vi "ProcessCurveData.vi"(11 "New Curve Values":T1) -> ()   [LabVIEW 2025]
uses:
  NewCurveDataEventArgs.ctl
  E:/PSCode/PalmSens_SDK/labview/PalmSens/Libraries/PalmSens.Core.Simplified.LabVIEW.dll
  Libraries/PalmSens.Core.Simplified.LabVIEW.dll
  LiveCurveResult.ctl
  MeasurementsResult.ctl
  MeasurementResults.ctl
  CurvesByMeasurement.ctl
  MeasurementInfo.ctl
  CurveInfo.ctl
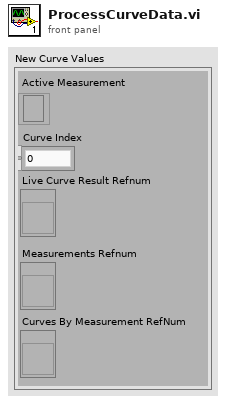
[diagram p1: front panel]
types:
  T1 = typedef "NewCurveDataEventArgs.ctl" = cluster{"Active Measurement":refnum<k24>, "Live Curve Result Refnum":refnum<vi>, "Measurements Refnum":refnum<vi>, "Curves By Measurement RefNum":refnum<vi>, "Curve Index":i32}
  T2 = typedef "CurvesByMeasurement.ctl" = map{refnum<k24>, T3}
  T3 = typedef "MeasurementInfo.ctl" = cluster{"Index":i32, "Is Measuring Refnum":refnum<vi>, "MeasurementEnded callback refnum":refnum<k27>, "SimpleCurveAdded callback refnum":refnum<k27>, "Live Curve Result Refnum":refnum<vi>, "Map":map{i32, T4}}
  T4 = typedef "CurveInfo.ctl" = cluster{"NewDataAdded callback refnum":refnum<k27>, "CurveFinished callback refnum":refnum<k27>}
  T5 = typedef "MeasurementsResult.ctl" = cluster{"Name":string, "Curves":T6, "Index":i32}[]
  T6 = typedef "MeasurementResults.ctl" = T7[]
  T7 = typedef "LiveCurveResult.ctl" = cluster{"X Label":string, "Y Label":string, "Name":string, "Index":i16, "Curve Values":cluster{"Values":cluster{"X Value":dbl, "Y Value":dbl}[], "Index":i16}}
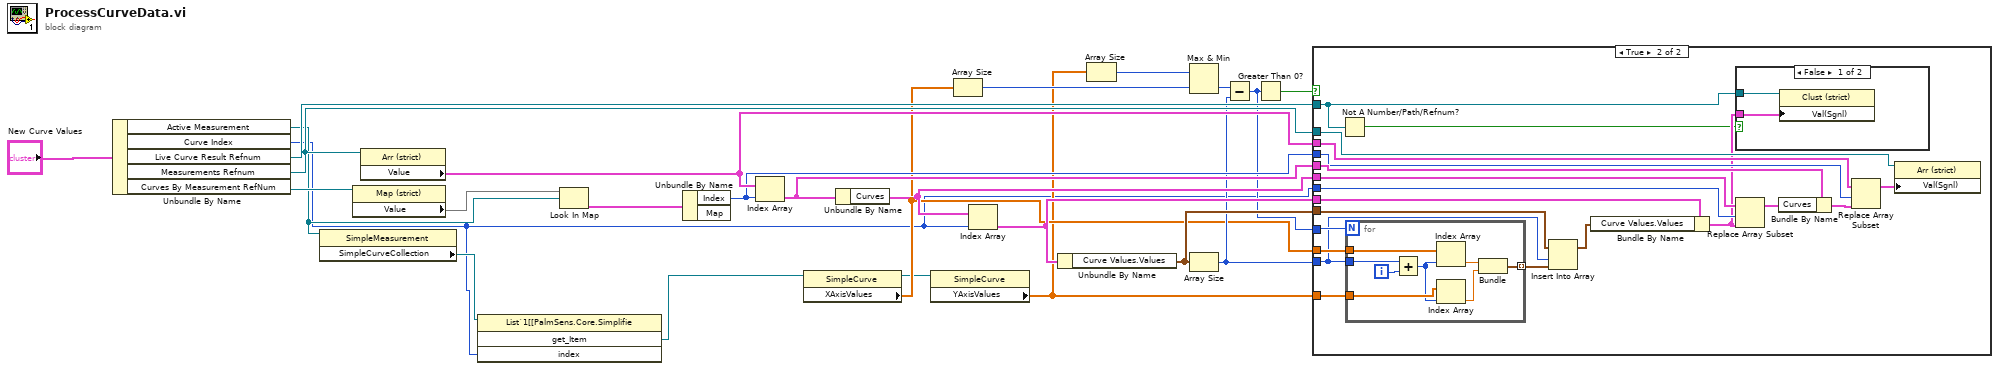
[diagram p0: block diagram]
diagram:
  n1 = Unbundle By Name("New Curve Values") -> ("Active Measurement"=w4:refnum<k24>, "Curve Index"=w2:i32, "Live Curve Result Refnum"=w21:refnum<vi>, "Measurements Refnum"=w25:refnum<vi>, "Curves By Measurement RefNum"=w9:refnum<vi>)
  n2 = property class="SimpleMeasurement"(reference=w4) -> ("SimpleCurveCollection"=w3:refnum<k24>)  [unwired: 1 in, 2 out]
  n3 = property class="Map (strict)"(reference=w9) -> ("Value"=w10:T2)  [unwired: 1 in, 2 out]
  n4 = property class="Arr (strict)"(reference=w25) -> ("Value"=w24:T5)  [unwired: 1 in, 2 out]
  n5 = invoke class="List`1[[PalmSens.Core.Simplifie" method="get_Item"(reference=w3, "index"=w2) -> ("get_Item"=w1:refnum<k24>)  [unwired: 2 in, 3 out]
  n6 = Look In Map(map=w10, key=w4) -> (value=w11:T3)  [unwired: 1 in, 1 out]
  n7 = Unbundle By Name(w11) -> ("Index"=w23:i32)  [unwired: 1 out]
  n8 = Index Array(array=w24, index=w23) -> (element=w22:cluster{"Name":string, "Curves":T6, "Index":i32})
  n9 = property class="SimpleCurve"(reference=w1) -> (reference out=w5:refnum<k24>, "XAxisValues"=w12:dbl[])  [unwired: 1 in, 1 out]
  n10 = Unbundle By Name(w22) -> ("Curves"=w20:T6)
  n11 = property class="SimpleCurve"(reference=w5) -> ("YAxisValues"=w7:dbl[])  [unwired: 1 in, 2 out]
  n12 = Array Size(array=w12) -> (size(s)=w13:i32)
  n13 = Index Array(array=w20, index=w2) -> (element=w19:T7)
  n14 = Unbundle By Name(w19) -> ("Curve Values.Values"=w18:cluster{"X Value":dbl, "Y Value":dbl}[])
  n15 = Array Size(array=w7) -> (size(s)=w6:i32)
  n16 = Max & Min(x=w6, y=w13) -> (min(x,y)=w14:i32)  [unwired: 1 out]
  n17 = Array Size(array=w18) -> (size(s)=w17:i32)
  n18 = Subtract(x=w14, y=w17) -> (x-y=w16:i32)
  n19 = Greater Than 0?(x=w16) -> (x > 0?=w15:bool)
  n20 = case shown="True" w15 {
    tunnel: w12 -> [_ w45]
    tunnel: w7 -> [_ w44]
    tunnel: w16 -> [_ w43]
    tunnel: w17 -> [_ w41]
    tunnel: w18 -> [_ w42]
    tunnel: w19 -> [_ w38]
    tunnel: w20 -> [_ w37]
    tunnel: w2 -> [_ w36]
    tunnel: w21 -> [_ w26]
    tunnel: w22 -> [_ w35]
    tunnel: w23 -> [_ w32]
    tunnel: w24 -> [_ w31]
    tunnel: w25 -> [_ w29]
    frame False {
    }
    frame True {
      n21 = Not A Number/Path/Refnum?(number/path/refnum=w26) -> (NaN/Path/Refnum?=w27:bool)
      n22 = for {
        N: w43 -> [_]
        tunnel: w45 -> [w55]
        tunnel: w44 -> [w52]
        tunnel: [w49] -> w40 mode=indexing
        tunnel: w41 -> [w48]
        i -> [w54]
        n23 = Add(x=w48, y=w54) -> (x+y=w51:i32)
        n24 = Index Array(array=w55, index=w51) -> (element=w53:dbl)
        n25 = Index Array(array=w52, index=w51) -> (element=w50:dbl)
        n26 = Bundle(w53, w50) -> (w49:cluster{dbl, dbl})  [unwired: 1 in]
      }
      n27 = Insert Into Array(array=w42, index=w41, new element=w40) -> (w39:cluster{"X Value":dbl, "Y Value":dbl}[])
      n28 = Bundle By Name(cluster=w38, "Curve Values.Values"=w39) -> (w28:T7)
      n29 = case shown="False" w27 {
        tunnel: w26 -> [w47 _]
        tunnel: w28 -> [w46 _]
        frame False {
          n30 = property class="Clust (strict)"(reference=w47, "Val(Sgnl)"=w46) -> ()  [unwired: 1 in, 2 out]
        }
        frame True {
        }
      }
      n31 = Replace Array Subset(array=w37, new element=w28, index=w36) -> (w34:T6)
      n32 = Bundle By Name(cluster=w35, "Curves"=w34) -> (w33:cluster{"Name":string, "Curves":T6, "Index":i32})
      n33 = Replace Array Subset(array=w31, new element=w33, index=w32) -> (w30:T5)
      n34 = property class="Arr (strict)"(reference=w29, "Val(Sgnl)"=w30) -> ()  [unwired: 1 in, 2 out]
    }
  }
